vi "GetType.vi"(8 "error in (no error)":errorcluster, 11 "Configure AC Bandwidth [AC] Msg":refnum<class "Configure AC Bandwidth [AC] Msg.lvclass">) -> (0 "error out":errorcluster, 2 "Data Sample":variant, 3 "Configure AC Bandwidth [AC] Msg":refnum<class "Configure AC Bandwidth [AC] Msg.lvclass">)   [LabVIEW 2015, in "CS++DMM.lvlib" / "Configure AC Bandwidth [AC] Msg.lvclass"]
uses:
  Configure AC Bandwidth [AC] Msg.lvclass
  Configure AC Bandwidth [AC] Msg.lvclass/Configure AC Bandwidth [AC] Msg.ctl
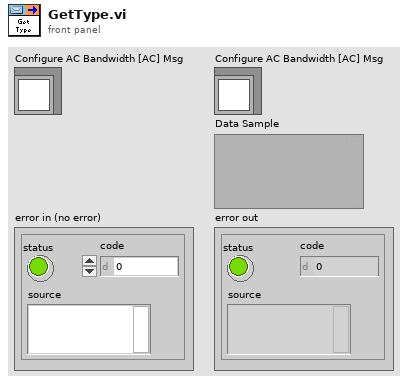
[diagram p1: front panel]
types:
  T1 = cluster{"ac min frequency (20.0 Hz)":dbl, "ac max frequency (300.0E+3 Hz)":dbl}
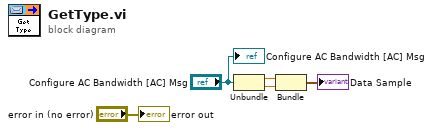
[diagram p0: block diagram]
diagram:
  n1 = Unbundle("Configure AC Bandwidth [AC] Msg") -> (w2:dbl, w1:dbl)
  n2 = Bundle("ac min frequency (20.0 Hz)"=w2, "ac max frequency (300.0E+3 Hz)"=w1) -> (→"Data Sample":T1)  [unwired: 1 in]
  "error out" <- "error in (no error)"
  "Configure AC Bandwidth [AC] Msg" <- "Configure AC Bandwidth [AC] Msg"
